vi "Get Object By ID.vi"(8 "error in (no error)":errorcluster, 10 "ID":i32=-1, 11 "Objects in":refnum<class "Objects.lvclass">) -> (0 "error out":errorcluster, 1 "Object":refnum<class "Object.lvclass">, 3 "Objects out":refnum<class "Objects.lvclass">)   [LabVIEW 2019, in "HierDAL Library.lvlib" / "Database.lvlib" / "Repositories.lvlib" / "Objects.lvclass"]
uses:
  Objects.lvclass
  Models Library/Object Class/Object.lvclass
  Objects.lvclass/Objects.ctl
  46314e7c-a004-450c-aec5-182bd9d357fe.vi
  Database Manager Class/Database Manager.lvclass
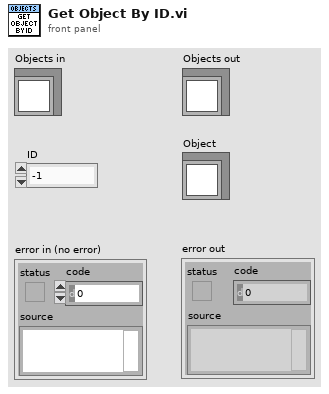
[diagram p1: front panel]
types:
  T1 = typedef "HierDAL Library.lvlib/Common.lvlib/Datatype.ctl" = enum16{"Unknown", "Group", "Dataset"}
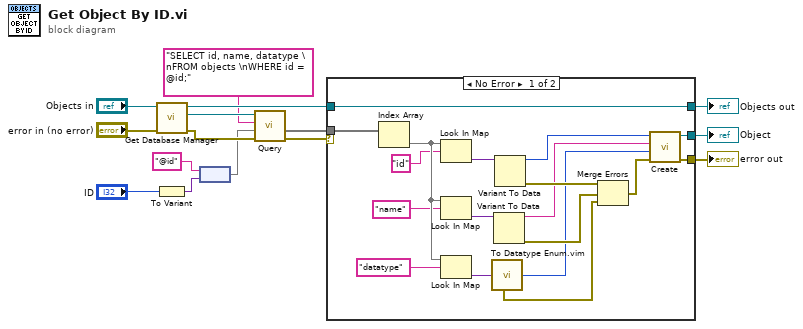
[diagram p0: block diagram]
diagram:
  n1 = call "Get Database Manager.vi"("error in (no error)"="error in (no error)", "Objects in"="Objects in") -> ("error out"=w14:errorcluster, "Database Manager"=w13:refnum<class "Database Manager.lvclass">, "Objects out"=w15:refnum<class "Objects.lvclass">)  [unwired: 7 in]
  n2 = To Variant(anything="ID") -> (Variant=w12:variant)
  n3 = node("@id" ("key"), w12) -> (w7:map{string, variant})
  n4 = call-dynamic "Query.vi"("error in (no error)"=w14, "Parameters"=w7, "Query"="SELECT id, name, datatype \nFROM objects \nWHERE id = @id;", "Database Manager in"=w13) -> ("error out"=w2:errorcluster, "Rows"=w4:map{string, variant}[])  [unwired: 5 in, 1 out]
  n5 = case shown="No Error" w2 {
    selector: w2 -> [_ w34]
    tunnel: [w32 _] -> w5
    tunnel: w4 -> [w31 _]
    tunnel: [w21 w34] -> w3
    tunnel: w15 -> [w20 w35]
    tunnel: [w20 w35] -> w1
    frame No Error {
      n6 = Index Array(array=w31) -> (element=w33:map{string, variant})  [unwired: 1 in]
      n7 = Look In Map(map=w33, key="id") -> (value=w27:variant)  [unwired: 1 in, 1 out]
      n8 = Look In Map(map=w33, key="name") -> (value=w25:variant)  [unwired: 1 in, 1 out]
      n9 = Look In Map(map=w33, key="datatype") -> (value=w18:variant)  [unwired: 1 in, 1 out]
      n10 = call "To Datatype Enum.vim"("Value"=w18) -> ("error out"=w17:errorcluster, "Datatype"=w16:T1)  [unwired: 5 in]
      n11 = Variant To Data(Variant=w25) -> (data=w19:string, error out=w23:errorcluster)  [unwired: 2 in]
      n12 = Variant To Data(Variant=w27) -> (data=w26:i32, error out=w24:errorcluster)  [unwired: 2 in]
      n13 = Merge Errors(w24, w23, w17) -> (w22:errorcluster)
      n14 = call "Create.vi"("error in (no error)"=w22, "Datatype"=w16, "Name"=w19, "ID"=w26) -> ("error out"=w21:errorcluster, "Object out"=w32:refnum<class "Object.lvclass">)  [unwired: 6 in]
    }
    frame Error {
    }
  }
  "error out" <- w3
  "Objects out" <- w1
  "Object" <- w5
